vi "Modify Selected Graphicvi.vi"(8 "error in (no error)":errorcluster, 9 "Coords":T1, 11 "Canvas in":refnum<class "Canvas.lvclass">) -> (0 "error out":errorcluster, 3 "Canvas out":refnum<class "Canvas.lvclass">)   [LabVIEW 2015, in "Canvas.lvclass"]
uses:
  Canvas.lvclass
  <vilib>/Utility/miscctls.llb/LVPoint32TypeDef.ctl
  Canvas.lvclass/Canvas.ctl
  Graphic/Graphic.lvclass/Graphic.ctl
  Scalable Border/Scalable Border.lvclass
  Graphic/Graphic.lvclass
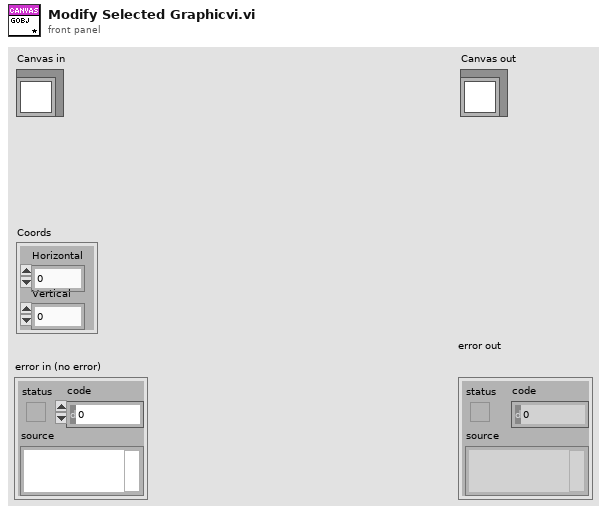
[diagram p1: front panel]
types:
  T1 = typedef "LVPoint32TypeDef.ctl" = cluster{"Horizontal":i32, "Vertical":i32}
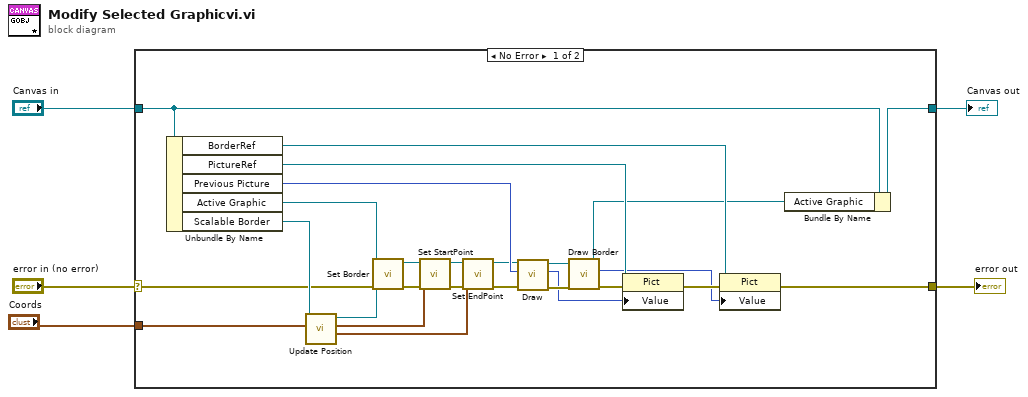
[diagram p0: block diagram]
diagram:
  n1 = case shown="No Error" "error in (no error)" {
    selector: "error in (no error)" -> [w11 w33]
    tunnel: [w16 w33] -> w4
    tunnel: [w15 w32] -> w2
    tunnel: "Canvas in" -> [w6 w32]
    tunnel: "Coords" -> [w30 _]
    frame No Error {
      n2 = Unbundle By Name(w6) -> ("BorderRef"=w14:refnum<vi>, "PictureRef"=w20:refnum<vi>, "Previous Picture"=w26:picture, "Active Graphic"=w9:refnum<class "Graphic.lvclass">, "Scalable Border"=w13:refnum<class "Scalable Border.lvclass">)
      n3 = call-dynamic "Update Position.vi"("Diff"=w30, "Scalable Border in"=w13) -> ("EndPoint"=w27:cluster{"x":i16, "y":i16}, "StartPoint"=w28:cluster{"x":i16, "y":i16}, "Scalable Border out"=w7:refnum<class "Scalable Border.lvclass">)  [unwired: 6 in, 1 out]
      n4 = call "Set Border.vi"("error in (no error)"=w11, "Scalable Border.lvclass"=w7, "Graphic in"=w9) -> ("error out"=w10:errorcluster, "Graphic out"=w8:refnum<class "Graphic.lvclass">)  [unwired: 7 in]
      n5 = call "Set StartPoint.vi"("error in (no error)"=w10, "StartPoint"=w28, "Graphic in"=w8) -> ("error out"=w24:errorcluster, "Graphic out"=w29:refnum<class "Graphic.lvclass">)  [unwired: 7 in]
      n6 = call "Set EndPoint.vi"("error in (no error)"=w24, "EndPoint"=w27, "Graphic in"=w29) -> ("error out"=w23:errorcluster, "Graphic out"=w25:refnum<class "Graphic.lvclass">)  [unwired: 7 in]
      n7 = call-dynamic "Draw.vi"("error in (no error)"=w23, "Picture in"=w26, "Graphic in"=w25) -> ("error out"=w22:errorcluster, "Picture out"=w19:picture, "Graphic out"=w31:refnum<class "Graphic.lvclass">)  [unwired: 6 in]
      n8 = call-dynamic "Draw Border.vi"("error in (no error)"=w22, "Graphic in"=w31) -> ("error out"=w21:errorcluster, "Picture out"=w17:picture, "Graphic out"=w12:refnum<class "Graphic.lvclass">)  [unwired: 7 in]
      n9 = property class="Pict"(reference=w20, error in=w21, "Value"=w19) -> (error out=w18:errorcluster)  [unwired: 1 out]
      n10 = property class="Pict"(reference=w14, error in=w18, "Value"=w17) -> (error out=w16:errorcluster)  [unwired: 1 out]
      n11 = Bundle By Name(cluster=w6, "Active Graphic"=w12) -> (w15:refnum<class "Canvas.lvclass">)
    }
    frame Error {
    }
  }
  "error out" <- w4
  "Canvas out" <- w2
